vi "Message_Read.vi"(0 "VISA in":refnum<visa-resource-name>, 5 "Message":u16(ring) items=["Warning", "FanPWM", "Temperature", "Humidity"], 11 "error in":errorcluster) -> (3 "Warning":bool, 4 "VISA out":refnum<visa-resource-name>, 6 "FanPWM":string, 8 "Tempature":string, 10 "Humidity":string, 15 "error out":errorcluster)   [LabVIEW 2019]
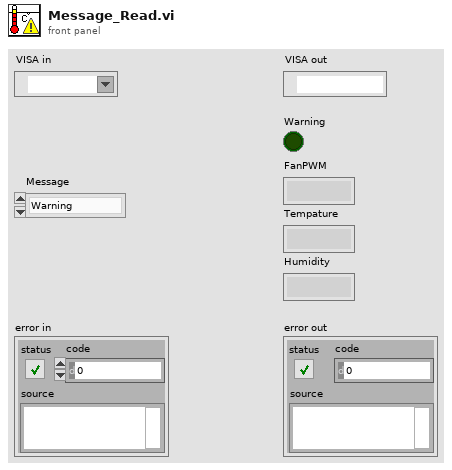
[diagram p1: front panel]
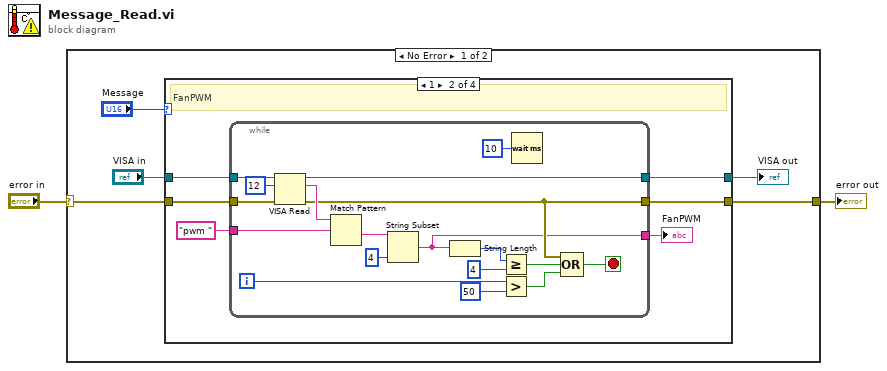
[diagram p0: block diagram]
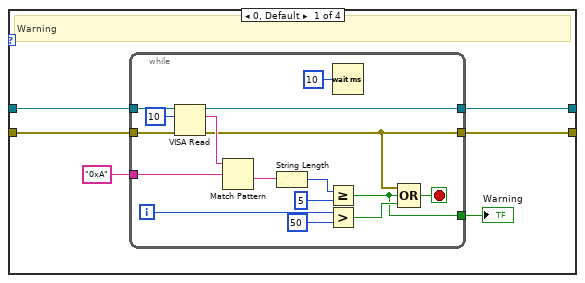
[diagram p2: hidden frame]
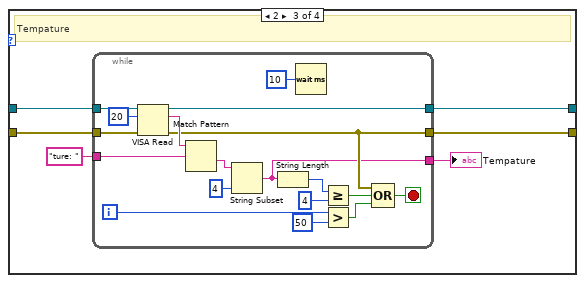
[diagram p3: hidden frame]
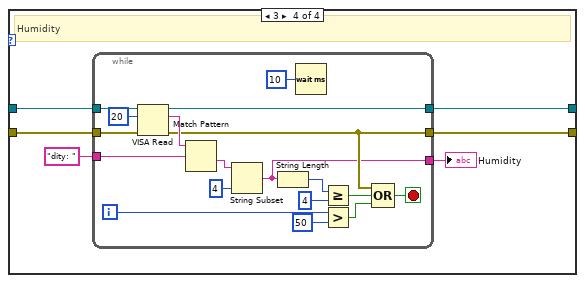
[diagram p4: hidden frame]
diagram:
  n1 = case shown="No Error" "error in" {
    selector: "error in" -> [w6 w102]
    tunnel: [w5 w102] -> w1
    frame No Error {
      n2 = case shown="1" "Message" {
        tunnel: "VISA in" -> [w13 w35 w59 w83]
        tunnel: w6 -> [w12 w34 w58 w82]
        tunnel: [w11 w33 w57 w81] -> w4
        tunnel: [w10 w32 w56 w80] -> w5
        frame 0, Default {
          # "Warning"
          n3 = while {
            tunnel: w13 -> [w28]
            tunnel: w12 -> [w27]
            tunnel: [w25] -> w11
            tunnel: [w19] -> w10
            tunnel: "0xA" ("regular expression") -> [w22]
            tunnel: [w14] -> w8
            i -> [w17]
            stop <- w18 stop-if-true
            n4 = VISA Read(VISA resource name=w28, byte count=u32 10, error in (no error)=w27) -> (VISA resource name out=w25:refnum<visa-resource-name>, read buffer=w26:string, error out=w19:errorcluster)  [unwired: 1 out]
            n5 = Match Pattern(string=w26, regular expression=w22) -> (after substring=w21:string)  [unwired: 1 in, 3 out]
            n6 = String Length(string=w21) -> (length=w24:i32)
            n7 = Greater Or Equal?(x=w24, y=5) -> (x >= y?=w14:bool)
            n8 = Greater?(x=w17, y=50) -> (0:w15:bool)
            n9 = Wait (ms)(milliseconds to wait=u32 10) -> ()  [unwired: 1 out]
            n10 = Compound Arithmetic op=OR(w19, w14, w15) -> (w18:bool)
          }
          "Warning" <- w8
        }
        frame 1 {
          # "FanPWM"
          n11 = while {
            tunnel: w35 -> [w52]
            tunnel: w34 -> [w51]
            tunnel: [w49] -> w33
            tunnel: [w44] -> w32
            tunnel: "pwm " ("regular expression") -> [w46]
            tunnel: [w36] -> w30
            i -> [w42]
            stop <- w43 stop-if-true
            n12 = VISA Read(VISA resource name=w52, byte count=u32 12, error in (no error)=w51) -> (VISA resource name out=w49:refnum<visa-resource-name>, read buffer=w50:string, error out=w44:errorcluster)  [unwired: 1 out]
            n13 = Match Pattern(string=w50, regular expression=w46) -> (after substring=w38:string)  [unwired: 1 in, 3 out]
            n14 = String Subset(string=w38, length (rest)=4 ("length (rest)")) -> (substring=w36:string)  [unwired: 1 in]
            n15 = String Length(string=w36) -> (length=w48:i32)
            n16 = Greater Or Equal?(x=w48, y=4) -> (x >= y?=w39:bool)
            n17 = Greater?(x=w42, y=50) -> (0:w40:bool)
            n18 = Wait (ms)(milliseconds to wait=u32 10) -> ()  [unwired: 1 out]
            n19 = Compound Arithmetic op=OR(w44, w39, w40) -> (w43:bool)
          }
          "FanPWM" <- w30
        }
        frame 2 {
          # "Tempature"
          n20 = while {
            tunnel: w59 -> [w76]
            tunnel: w58 -> [w75]
            tunnel: [w73] -> w57
            tunnel: [w68] -> w56
            tunnel: "ture: " ("regular expression") -> [w70]
            tunnel: [w60] -> w54
            i -> [w66]
            stop <- w67 stop-if-true
            n21 = VISA Read(VISA resource name=w76, byte count=u32 20, error in (no error)=w75) -> (VISA resource name out=w73:refnum<visa-resource-name>, read buffer=w74:string, error out=w68:errorcluster)  [unwired: 1 out]
            n22 = Match Pattern(string=w74, regular expression=w70) -> (after substring=w61:string)  [unwired: 1 in, 3 out]
            n23 = String Subset(string=w61, length (rest)=4 ("length (rest)")) -> (substring=w60:string)  [unwired: 1 in]
            n24 = String Length(string=w60) -> (length=w72:i32)
            n25 = Wait (ms)(milliseconds to wait=u32 10) -> ()  [unwired: 1 out]
            n26 = Greater Or Equal?(x=w72, y=4) -> (x >= y?=w63:bool)
            n27 = Greater?(x=w66, y=50) -> (0:w64:bool)
            n28 = Compound Arithmetic op=OR(w68, w63, w64) -> (w67:bool)
          }
          "Tempature" <- w54
        }
        frame 3 {
          # "Humidity"
          n29 = while {
            tunnel: w83 -> [w100]
            tunnel: w82 -> [w99]
            tunnel: [w97] -> w81
            tunnel: [w92] -> w80
            tunnel: "dity: " ("regular expression") -> [w94]
            tunnel: [w84] -> w78
            i -> [w90]
            stop <- w91 stop-if-true
            n30 = VISA Read(VISA resource name=w100, byte count=u32 20, error in (no error)=w99) -> (VISA resource name out=w97:refnum<visa-resource-name>, read buffer=w98:string, error out=w92:errorcluster)  [unwired: 1 out]
            n31 = Match Pattern(string=w98, regular expression=w94) -> (after substring=w85:string)  [unwired: 1 in, 3 out]
            n32 = String Subset(string=w85, length (rest)=4 ("length (rest)")) -> (substring=w84:string)  [unwired: 1 in]
            n33 = String Length(string=w84) -> (length=w96:i32)
            n34 = Wait (ms)(milliseconds to wait=u32 10) -> ()  [unwired: 1 out]
            n35 = Greater Or Equal?(x=w96, y=4) -> (x >= y?=w87:bool)
            n36 = Greater?(x=w90, y=50) -> (0:w88:bool)
            n37 = Compound Arithmetic op=OR(w92, w87, w88) -> (w91:bool)
          }
          "Humidity" <- w78
        }
      }
      "VISA out" <- w4
    }
    frame Error {
    }
  }
  "error out" <- w1
